vi "SwerveShortestTurnAlg.vi"(8 "SwerveMotorsFlipped?":bool, 9 "SwerveSpeed":dbl, 10 "AngleSetpoint":dbl, 11 "AngleEncoder":dbl) -> (2 "FlipSwerveMotors":bool, 3 "PIDInput":dbl)   [LabVIEW 2018]
uses:
  SwerveGlobals.vi
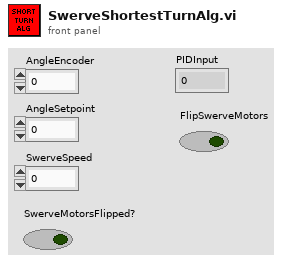
[diagram p1: front panel]
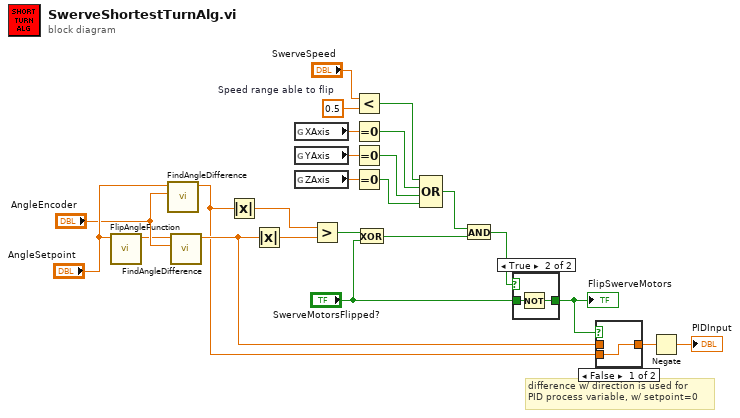
[diagram p0: block diagram]
diagram:
  w16 = 0.5  # Speed range able to flip
  # "difference w/ direction is used for\nPID process variable, w/ setpoint=0"
  n1 = call "FlipAngleFunction.vi"("AngleInput"="AngleSetpoint") -> ("AngleFlipped"=w18:dbl)  [unwired: 10 in]
  n2 = call "FindAngleDifference.vi"("AngleEncoder"="AngleEncoder", "AngleSetpoint"="AngleSetpoint") -> ("Distance/DirectionOfTurn"=w17:dbl)  [unwired: 9 in]
  n3 = call "FindAngleDifference.vi"("AngleEncoder"="AngleEncoder", "AngleSetpoint"=w18) -> ("Distance/DirectionOfTurn"=w19:dbl)  [unwired: 9 in]
  n4 = Absolute Value(x=w17) -> (abs(x)=w11:dbl)
  n5 = Absolute Value(x=w19) -> (abs(x)=w10:dbl)
  n6 = global read "SwerveGlobals.vi" "XAxis"() -> (w6:dbl)
  n7 = global read "SwerveGlobals.vi" "YAxis"() -> (w8:dbl)
  n8 = global read "SwerveGlobals.vi" "ZAxis"() -> (w15:dbl)
  n9 = Greater?(x=w11, y=w10) -> (0:w13:bool)
  n10 = Less?(x="SwerveSpeed", y=w16) -> (x < y?=w4:bool)
  n11 = Equal To 0?(x=w6) -> (x = 0?=w5:bool)
  n12 = Equal To 0?(x=w8) -> (x = 0?=w7:bool)
  n13 = Equal To 0?(x=w15) -> (x = 0?=w9:bool)
  n14 = Exclusive Or(1:"SwerveMotorsFlipped?", 2:w13) -> (0:w3:bool)
  n15 = Compound Arithmetic op=OR(w4, w5, w7, w9) -> (w1:bool)
  n16 = And(x=w1, y=w3) -> (x .and. y?=w2:bool)
  n17 = case shown="True" w2 {
    tunnel: "SwerveMotorsFlipped?" -> [w25 w27]
    tunnel: [w25 w26] -> w21
    frame False {
    }
    frame True {
      n18 = Not(x=w27) -> (.not. x?=w26:bool)
    }
  }
  "FlipSwerveMotors" <- w21
  n19 = case shown="False" w21 {
    tunnel: w17 -> [w28 _]
    tunnel: w19 -> [_ w29]
    tunnel: [w28 w29] -> w20
    frame False {
    }
    frame True {
    }
  }
  n20 = Negate(x=w20) -> (-x=→"PIDInput":dbl)
